vi "Create Mask By Alpha - Advanced -__jki_lib_picture -- VI Tester.vi"(9 "Background color (White)":u32(colorbox)=16777215, 10 "Transparency Thresh":u8=127, 11 "image data":T1) -> (3 "masked image data":T1)   [LabVIEW 2011]
uses:
  <vilib>/picture/picture.llb/imagedata.ctl
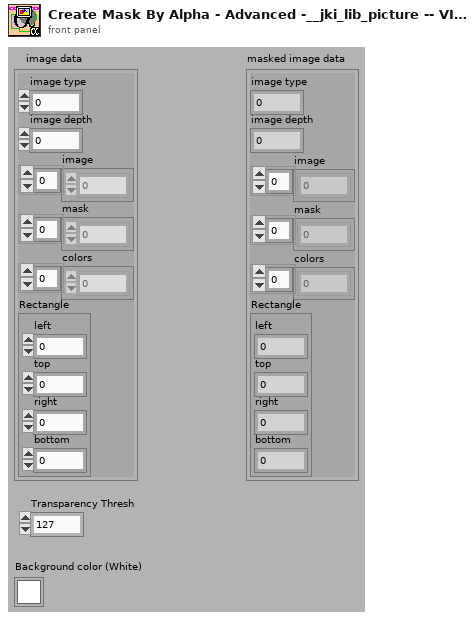
[diagram p1: front panel]
types:
  T1 = typedef "imagedata.ctl" = cluster{"image type":i32, "image depth":i32, "image":u8[], "mask":u8[], "colors":u32[], "Rectangle":cluster{"left":i16, "top":i16, "right":i16, "bottom":i16}}
  T2 = cluster{"left":i16, "top":i16, "right":i16, "bottom":i16}
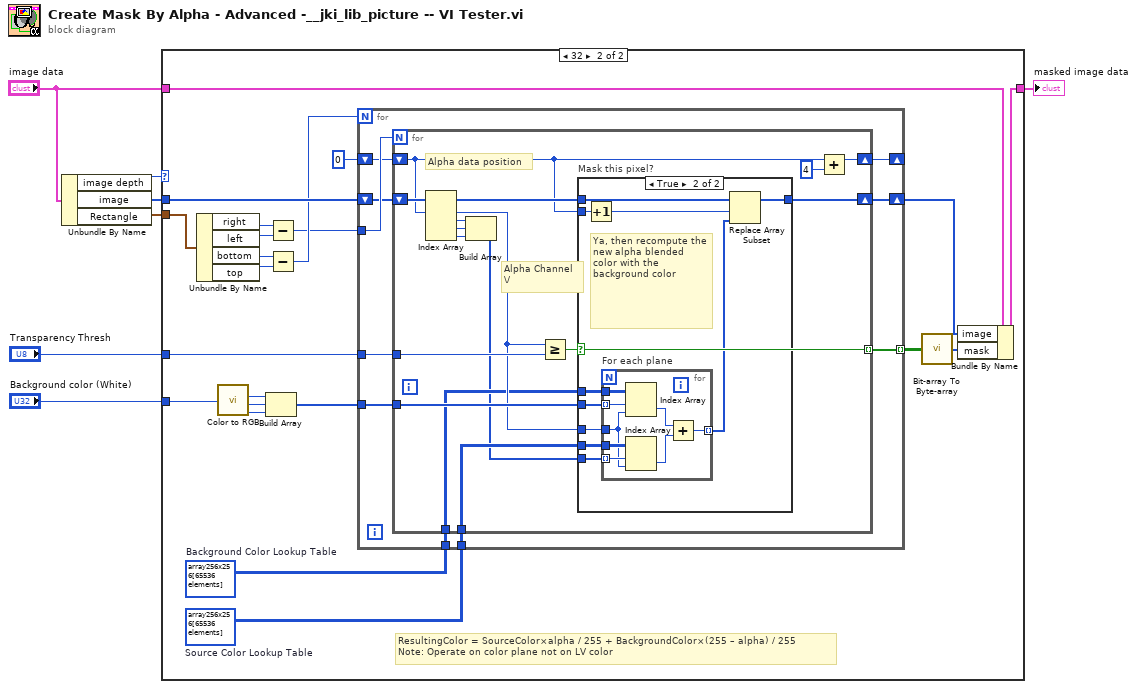
[diagram p0: block diagram]
diagram:
  n1 = Unbundle By Name("image data") -> ("image depth"=w7:i32, "image"=w5:u8[], "Rectangle"=w6:T2)
  n2 = case shown="32" w7 {
    tunnel: w6 -> [_ w30]
    tunnel: w5 -> [_ w25]
    tunnel: "image data" -> [w8 w21]
    tunnel: [w8 w20] -> w3
    tunnel: "Background color (White)" -> [_ w15]
    tunnel: "Transparency Thresh" -> [_ w16]
    frame Default {
    }
    frame 32 {
      w10 = u8[][] array256x256[65536 elements]  # Source Color Lookup Table
      w17 = u8[][] array256x256[65536 elements]  # Background Color Lookup Table
      # "ResultingColor = SourceColor×alpha / 255 + BackgroundColor×(255 – alpha) / 255 \nNote: Operate on color plane not on LV color"
      n3 = Unbundle By Name(w30) -> ("right"=w29:i16, "left"=w28:i16, "bottom"=w27:i16, "top"=w26:i16)
      n4 = call <vilib>:"Color to RGB.vi"("Color"=w15) -> ("R"=w14:u8, "G"=w13:u8, "B"=w12:u8)  [unwired: 1 out]
      n5 = Build Array(w14, w13, w12) -> (w11:u8[])
      n6 = Subtract(x=w29, y=w28) -> (x-y=w18:i16)
      n7 = Subtract(x=w27, y=w26) -> (x-y=w19:i16)
      n8 = for {
        N: w19 -> [_]
        tunnel: w18 -> [w40]
        shift-right: [w37] -> _
        shift-left: 0 -> [w38]
        tunnel: [w36] -> w23 mode=indexing
        tunnel: w17 -> [w35]
        tunnel: w16 -> [w34]
        tunnel: w11 -> [w33]
        tunnel: w10 -> [w32]
        shift-right: [w31] -> w9
        shift-left: w25 -> [w39]
        n9 = for {
          N: w40 -> [_]
          shift-right: [w55] -> w37
          shift-left: w38 -> [w41]
          tunnel: [w44] -> w36 mode=indexing
          tunnel: w35 -> [w50]
          tunnel: w34 -> [w53]
          tunnel: w33 -> [w52]
          tunnel: w32 -> [w49]
          shift-right: [w42] -> w31
          shift-left: w39 -> [w43]
          # "Alpha data position"
          # "Alpha Channel\n\\/"
          n10 = Index Array(array=w43, index #1=w41) -> (element #1=w51:u8, element #2=w48:u8, element #3=w47:u8, element #4=w46:u8)  [unwired: 3 in]
          n11 = Build Array(w48, w47, w46) -> (w45:u8[])
          n12 = Greater Or Equal?(x=w51, y=w53) -> (x >= y?=w44:bool)
          n13 = case "Mask this pixel?" shown="True" w44 {
            tunnel: w52 -> [_ w66]
            tunnel: w51 -> [_ w65]
            tunnel: w50 -> [_ w64]
            tunnel: w49 -> [_ w63]
            tunnel: w45 -> [_ w62]
            tunnel: w43 -> [w56 w61]
            tunnel: [w56 w57] -> w42
            tunnel: w41 -> [_ w60]
            frame False {
            }
            frame True {
              # "Ya, then recompute the new alpha blended color with the background color"
              n14 = Increment(x=w60) -> (x+1=w59:i32)
              n15 = for "For each plane" {
                tunnel: w66 -> [w73] mode=indexing
                tunnel: w62 -> [w71] mode=indexing
                tunnel: w64 -> [w74]
                tunnel: w63 -> [w72]
                tunnel: [w68] -> w58 mode=indexing
                tunnel: w65 -> [w67]
                n16 = Index Array(array=w74, index (row)=w73, index (col)=w67) -> (element=w70:u8)
                n17 = Index Array(array=w72, index (row)=w71, index (col)=w67) -> (element=w69:u8)
                n18 = Add(x=w70, y=w69) -> (x+y=w68:u8)
              }
              n19 = Replace Array Subset(array=w61, new element=w58, index=w59) -> (w57:u8[])
            }
          }
          n20 = Add(x=w41, y=4) -> (x+y=w55:i32)
        }
      }
      n21 = call <vilib>:"Bit-array To Byte-array.vi"("bit array"=w23) -> ("byte array"=w22:u8[])
      n22 = Bundle By Name(cluster=w21, "image"=w9, "mask"=w22) -> (w20:T1)
    }
  }
  "masked image data" <- w3
